vi "Calculate Average Sector Background.vi"(8 "error in (no error)":errorcluster, 9 "Image":T1, 10 "Right Sector Parameters":T3, 11 "Left Sector Parameters":T3) -> (0 "error out":errorcluster, 3 "[Avg BG]":dbl[](array[numeric]))   [LabVIEW 2013]
uses:
  FPGA/Sector/Accumulate/Sector Parameter Cluster.ctl
  FPGA/Sector/Accumulate/Accumulated Sector Cluster.ctl
  <vilib>/vision/Image Controls.llb/IMAQ Image.ctl
panel:
  out "Accumulated BG":T2[](array[typedef])
  # "Calculating Average Sector Background ..."
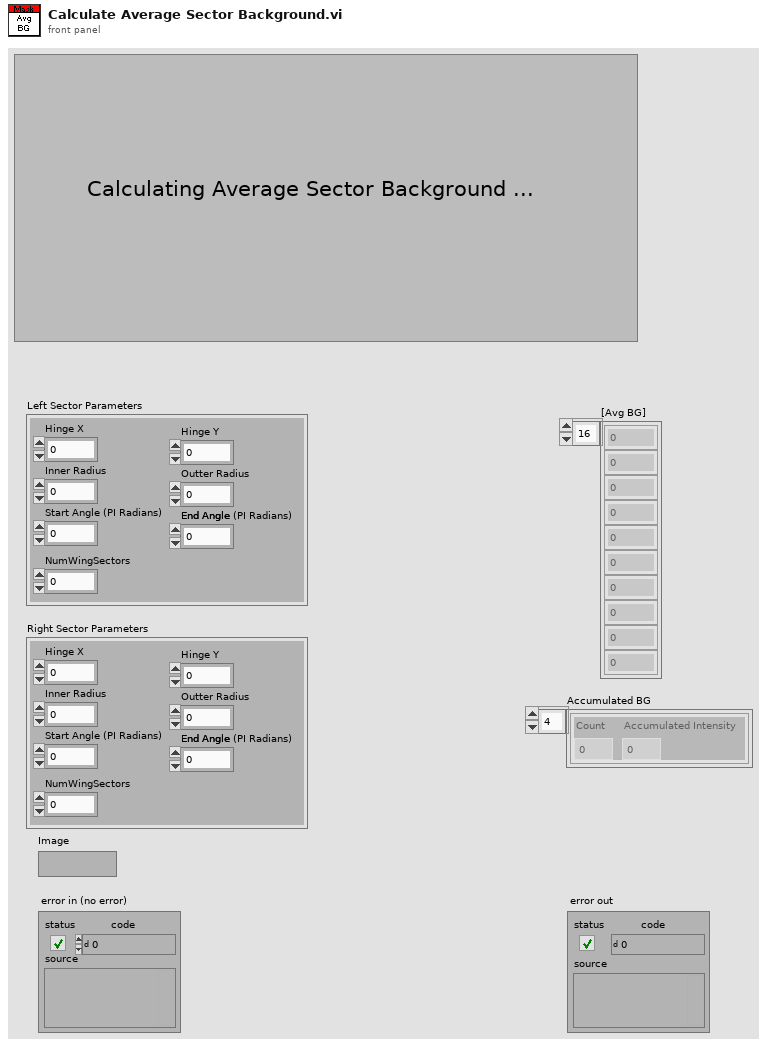
[diagram p1: front panel]
types:
  T1 = typedef "IMAQ Image.ctl" = refnum<image>
  T2 = typedef "Accumulated Sector Cluster.ctl" = cluster{"Accumulated Intensity":u32, "Count":u16}
  T3 = typedef "Sector Parameter Cluster.ctl" = cluster{"Start Angle":fxp<+,17,3>, "End Angle":fxp<+,17,3>, "Inner Radius":u16, "Outter Radius":u16, "Hinge X":u16, "Hinge Y":u16, "NumWingSectors":u8}
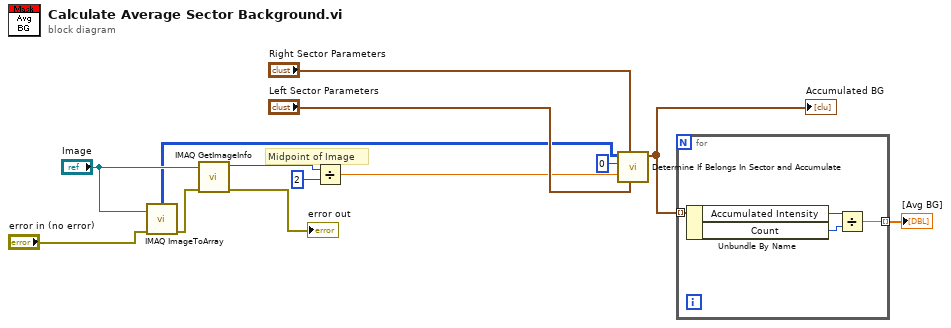
[diagram p0: block diagram]
diagram:
  # "Midpoint of Image"
  n1 = call "IMAQ ImageToArray"("error in (no error)"="error in (no error)", "Image"="Image") -> ("error out"=w4:errorcluster, "Image Pixels (U8)"=w2:u8[][])  [unwired: 2 in, 3 out]
  n2 = call "IMAQ GetImageInfo"("error in (no error)"=w4, "Image"="Image") -> ("error out"=→"error out":errorcluster, "X Resolution"=w13:i32)  [unwired: 2 in, 6 out]
  n3 = Divide(x=w13, y=2) -> (x/y=w8:dbl)
  n4 = call "Determine If Belongs In Sector and Accumulate.vi"("Left Sector Parameters"="Left Sector Parameters", "Right Sector Parameters"="Right Sector Parameters", "Midpoint of Image"=w8, "Starting Y Location"=0, "Image Data"=w2) -> ("[Accumulated Sectors]"=w1:T2[])  [unwired: 5 in, 1 out]
  "Accumulated BG" <- w1
  n5 = for {
    tunnel: w1 -> [w17] mode=indexing
    tunnel: [w14] -> w7 mode=indexing
    n6 = Unbundle By Name(w17) -> ("Accumulated Intensity"=w16:u32, "Count"=w15:u16)
    n7 = Divide(x=w16, y=w15) -> (x/y=w14:dbl)
  }
  "[Avg BG]" <- w7
